vi "GetType.vi"(8 "error in (no error)":errorcluster, 11 "Send Software Hold Trigger [HT] Msg":refnum<class "Send Software Hold Trigger [HT] Msg.lvclass">) -> (0 "error out":errorcluster, 2 "Data Sample":variant, 3 "Send Software Hold Trigger [HT] Msg":refnum<class "Send Software Hold Trigger [HT] Msg.lvclass">)   [LabVIEW 2015, in "CS++Fgen.lvlib" / "Send Software Hold Trigger [HT] Msg.lvclass"]
doc: "This VI delivers a sample of the data type format the message expects."
uses:
  Send Software Hold Trigger [HT] Msg.lvclass
  Send Software Hold Trigger [HT] Msg.lvclass/Send Software Hold Trigger [HT] Msg.ctl
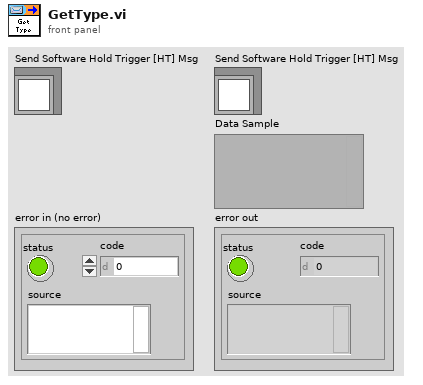
[diagram p1: front panel]
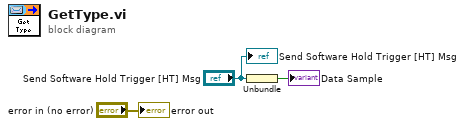
[diagram p0: block diagram]
diagram:
  n1 = Unbundle("Send Software Hold Trigger [HT] Msg") -> (→"Data Sample":bool)
  "error out" <- "error in (no error)"
  "Send Software Hold Trigger [HT] Msg" <- "Send Software Hold Trigger [HT] Msg"
